vi "Index uebersetzen.vi"(6 "Aktion":T3, 11 "Array":i32[][](array[numeric])) -> (2 "Komponenten":i32[](array[numeric]), 3 "Komponenten":T1 caption="Cluster")   [LabVIEW 2020, in "EPA 1065.lvlib" / "Interference verificaton 1065-375.lvlib"]
uses:
  Interference verificaton 1065-375.lvlib
  Aktion Index uebersetzten.ctl
  Komponenten.ctl
  Visualisierungs Elemente/String - Ausgabefeld.ctl
  Seiten/FT-IR/FGV FT-IR Gasliste Aktionen.ctl
  Aktion FGV Interference.ctl
  Seiten/FT-IR/FT-IR.lvlib
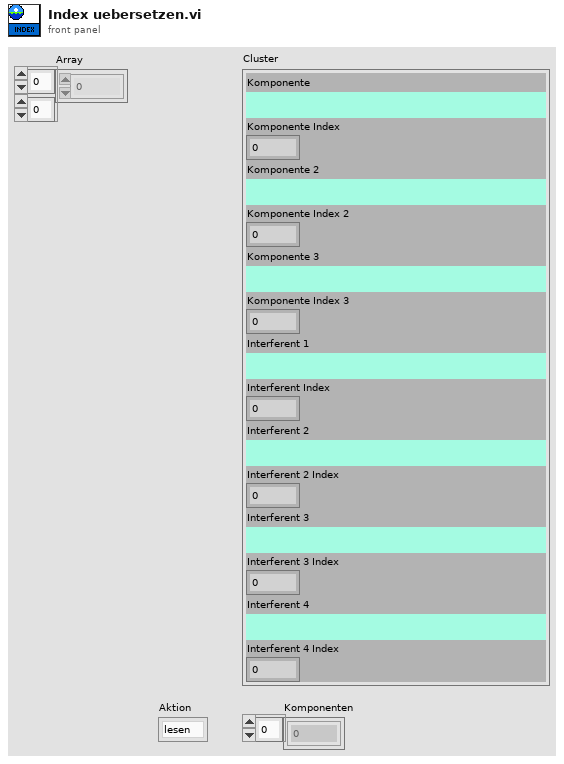
[diagram p1: front panel]
types:
  T1 = typedef "EPA 1065.lvlib/Interference verificaton 1065-375.lvlib/Komponenten.ctl" = cluster{"Komponente":T2, "Komponente Index":i32, "Komponente 2":T2, "Komponente Index 2":i32, "Komponente 3":T2, "Komponente Index 3":i32, "Interferent 1":T2, "Interferent Index":i32, "Interferent 2":T2, "Interferent 2 Index":i32, "Interferent 3":T2, "Interferent 3 Index":i32, "Interferent 4":T2, "Interferent 4 Index":i32}
  T2 = typedef "String - Ausgabefeld.ctl" = string
  T3 = typedef "EPA 1065.lvlib/Interference verificaton 1065-375.lvlib/Aktion Index uebersetzten.ctl" = enum16{"lesen", "schreiben", "auswerten"}
  T4 = typedef "EPA 1065.lvlib/Interference verificaton 1065-375.lvlib/Aktion FGV Interference.ctl" = enum16{"Lesen", "TestKonfig", "TestSetting", "Einheiten", "Ergebnis", "Laden", "Tabelle", "Speichern", "löschen"}
  T5 = typedef "FT-IR.lvlib/FGV FT-IR Gasliste Aktionen.ctl" = enum16{"lesen", "Gasliste FT-IR", "Gasliste ausgelesen", "laden", "speichern", "löschen"}
  T6 = typedef "EPA 1065.lvlib/Interference verificaton 1065-375.lvlib/TestKonfig.ctl" = cluster{"Komponente:":u16, "Modus":T7, "CG Aufschaltzeit:":dbl, "Interferent 1:":u16, "Interferent 2:":u16, "Interferent 3:":u16, "Gasflaschen Nr.:":string, "Gasflaschen Nr.: 2":string, "Gasflaschen Nr.: 3":string, "Inter 1 aktiv":bool, "Inter 2 aktiv":bool, "Inter 3 aktiv":bool, "Accuracy":string, "Accuracy 2":string, "Accuracy 3":string, "Konzentration 1:":dbl, "Konzentration 2:":dbl, "Konzentration 3:":dbl}
  T7 = typedef "EPA 1065.lvlib/Interference verificaton 1065-375.lvlib/Modus.ctl" = u16
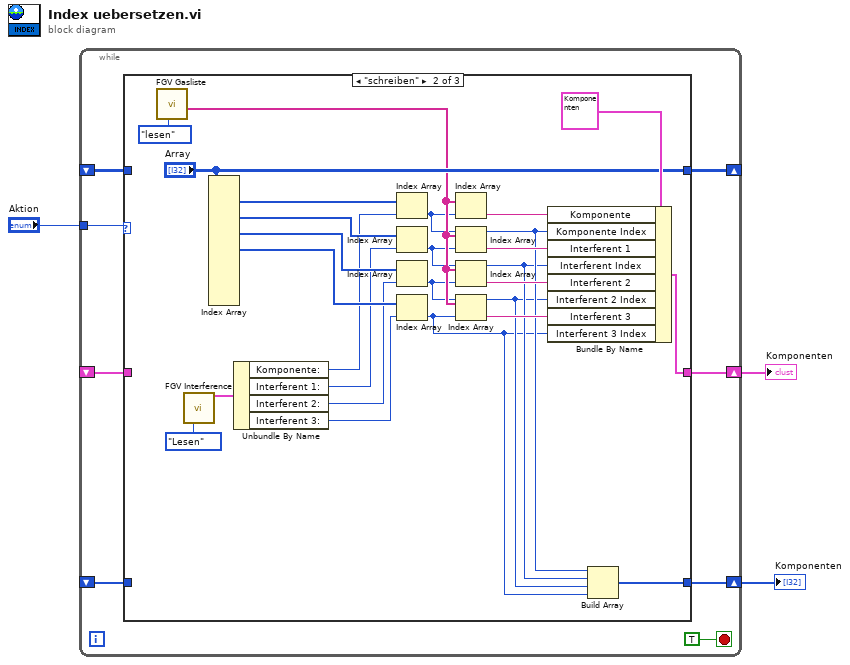
[diagram p0: block diagram]
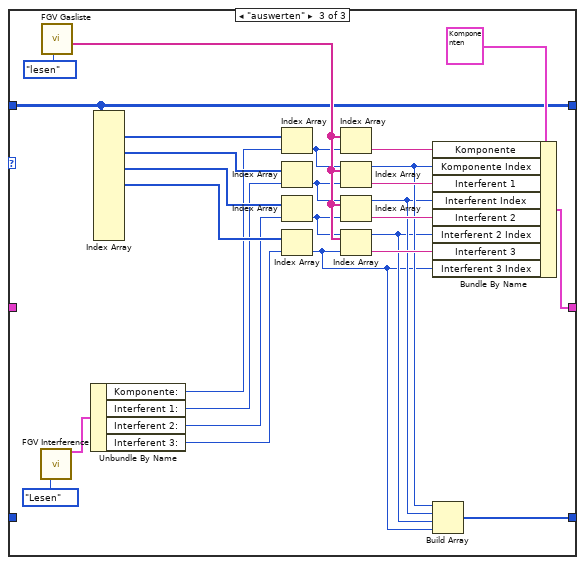
[diagram p3: hidden frame]
diagram:
  n1 = while {
    tunnel: "Aktion" -> [w10]
    shift-right: [w9] -> w2
    shift-left: _ -> [w8]
    shift-right: [w7] -> _
    shift-left: _ -> [w6]
    shift-right: [w5] -> w1
    shift-left: _ -> [w4]
    stop <- TRUE stop-if-true
    n2 = case shown="\"schreiben\"" w10 {
      tunnel: [w14 w34 w58] -> w9
      tunnel: w8 -> [w14 _ _]
      tunnel: [w12 "Array" w44] -> w7
      tunnel: w6 -> [w12 _ w44]
      tunnel: [w13 w19 w45] -> w5
      tunnel: w4 -> [w13 _ _]
      frame "lesen", Default {
      }
      frame "schreiben" {
        n3 = call "FGV Gasliste.vi"("Aktionen"=FGV_FT-IR_Gasliste_Aktionen."lesen") -> ("Aktuelle Gasliste gesamt"=w29:T2[])  [unwired: 8 in, 2 out]
        n4 = call "FGV Interference.vi"("Aktion FGV Interference"=Aktion_FGV_Interference."Lesen") -> ("TestKonfig 2"=w38:T6)  [unwired: 9 in, 5 out]
        n5 = Index Array(array="Array") -> (element #1=w32:i32[], element #2=w30:i32[], element #3=w26:i32[], element #4=w24:i32[])  [unwired: 14 in, 3 out]
        n6 = Unbundle By Name(w38) -> ("Komponente:"=w23:u16, "Interferent 1:"=w22:u16, "Interferent 2:"=w21:u16, "Interferent 3:"=w20:u16)
        n7 = Index Array(array=w32, index=w23) -> (element=w18:i32)
        n8 = Index Array(array=w30, index=w22) -> (element=w17:i32)
        n9 = Index Array(array=w26, index=w21) -> (element=w16:i32)
        n10 = Index Array(array=w24, index=w20) -> (element=w15:i32)
        n11 = Index Array(array=w29, index=w18) -> (element=w31:T2)
        n12 = Index Array(array=w29, index=w17) -> (element=w28:T2)
        n13 = Index Array(array=w29, index=w16) -> (element=w27:T2)
        n14 = Index Array(array=w29, index=w15) -> (element=w25:T2)
        n15 = Bundle By Name(cluster=T1 {"Komponente"="", "Komponente Index"=0, "Komponente 2"="", "Komponente Index 2"=0, "Komponente 3"="", "Komponente Index 3"=0, "Interferent 1"="", "Interferent Index"=0, "Interferent 2"="", "Interferent 2 Index"=0, "Interferent 3"="", "Interferent 3 Index"=0, "Interferent 4"="", "Interferent 4 Index"=0} ("Komponenten"), "Komponente"=w31, "Komponente Index"=w18, "Interferent 1"=w28, "Interferent Index"=w17, "Interferent 2"=w27, "Interferent 2 Index"=w16, "Interferent 3"=w25, "Interferent 3 Index"=w15) -> (w34:T1)
        n16 = Build Array(w18, w17, w16, w15) -> (w19:i32[])
      }
      frame "auswerten" {
        n17 = call "FGV Interference.vi"("Aktion FGV Interference"=Aktion_FGV_Interference."Lesen") -> ("TestKonfig 2"=w62:T6)  [unwired: 9 in, 5 out]
        n18 = call "FGV Gasliste.vi"("Aktionen"=FGV_FT-IR_Gasliste_Aktionen."lesen") -> ("Aktuelle Gasliste gesamt"=w54:T2[])  [unwired: 8 in, 2 out]
        n19 = Unbundle By Name(w62) -> ("Komponente:"=w42:u16, "Interferent 1:"=w41:u16, "Interferent 2:"=w40:u16, "Interferent 3:"=w39:u16)
        n20 = Index Array(array=w44) -> (element #1=w57:i32[], element #2=w55:i32[], element #3=w51:i32[], element #4=w49:i32[])  [unwired: 14 in, 3 out]
        n21 = Index Array(array=w57, index=w42) -> (element=w48:i32)
        n22 = Index Array(array=w55, index=w41) -> (element=w47:i32)
        n23 = Index Array(array=w51, index=w40) -> (element=w46:i32)
        n24 = Index Array(array=w49, index=w39) -> (element=w43:i32)
        n25 = Index Array(array=w54, index=w48) -> (element=w56:T2)
        n26 = Index Array(array=w54, index=w47) -> (element=w53:T2)
        n27 = Index Array(array=w54, index=w46) -> (element=w52:T2)
        n28 = Index Array(array=w54, index=w43) -> (element=w50:T2)
        n29 = Bundle By Name(cluster=T1 {"Komponente"="", "Komponente Index"=0, "Komponente 2"="", "Komponente Index 2"=0, "Komponente 3"="", "Komponente Index 3"=0, "Interferent 1"="", "Interferent Index"=0, "Interferent 2"="", "Interferent 2 Index"=0, "Interferent 3"="", "Interferent 3 Index"=0, "Interferent 4"="", "Interferent 4 Index"=0} ("Komponenten"), "Komponente"=w56, "Komponente Index"=w48, "Interferent 1"=w53, "Interferent Index"=w47, "Interferent 2"=w52, "Interferent 2 Index"=w46, "Interferent 3"=w50, "Interferent 3 Index"=w43) -> (w58:T1)
        n30 = Build Array(w48, w47, w46, w43) -> (w45:i32[])
      }
    }
  }
  "Komponenten" <- w2
  "Komponenten" <- w1
